vi "Globale Variablen Torque.vi"() -> ()   [LabVIEW 2018]
panel:
  out "Stop after measurement":bool
  out "Command-File":string
  out "Abbruchbedingung Messdauer":bool
  out "Zeiten für variable Temperatur final":dbl[](array[numeric])
  out "Zeiten für variables Magnetfeld final":dbl[](array[numeric])
  out "Fehler im Command-File":bool
  out "Ausgelesener Winkel":dbl
  in  "Winkel":dbl
  in  "Nur Position auslesen":bool
  out "Gesamtzeiten":dbl[](array[numeric])
  out "Zeiten für variables Magnetfeld init":dbl[](array[numeric])
  out "Messdaten":dbl[][](array[numeric])
  out "Zeiten für variable Temperatur init":dbl[](array[numeric])
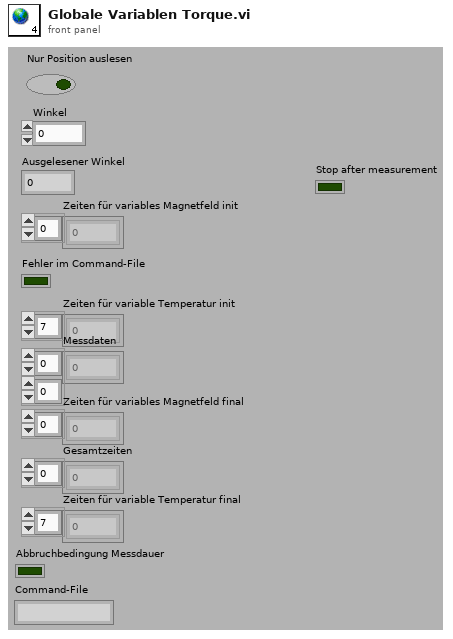
[diagram p1: front panel]
diagram:
